vi "get_counter_data.vi"(0 "Counter Settings, Tasks and Data (in)":T1, 5 "error in":errorcluster) -> (14 "Counter Settings, Tasks and Data":T1, 19 "error out":errorcluster)   [LabVIEW 2013]
uses:
  <vilib>/DAQmx/read.llb/DAQmx Read (Counter 1D U32 1Chan NSamp).vi
  <vilib>/DAQmx/miscellaneous.llb/DAQmx Fill In Error Info.vi
panel:
  out "counter data":u32[][](array[numeric])
  out "Last Counters Value":u32[](array[numeric])
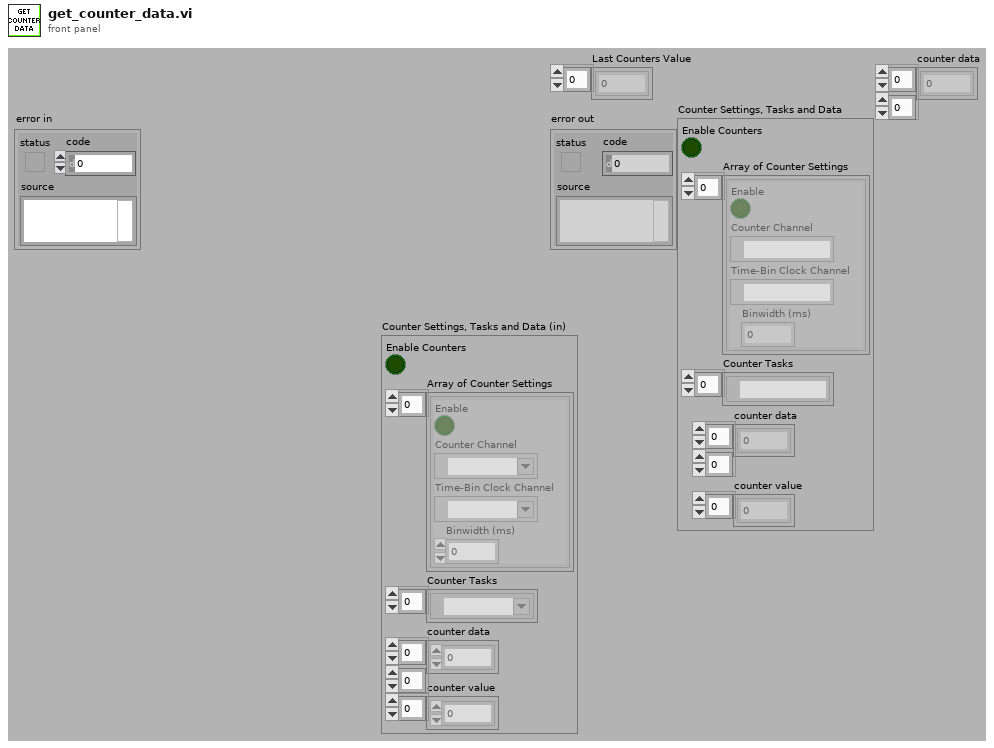
[diagram p1: front panel]
types:
  T1 = cluster{"Enable Counters":bool, "Array of Counter Settings":cluster{"Enable":bool, "Counter Channel":tag, "Time-Bin Clock Channel":tag, "Binwidth (ms)":dbl}[], "Counter Tasks":refnum<k21>[], "counter data":u32[][], "counter value":u32[]}
  T2 = cluster{"Enable":bool, "Counter Channel":tag, "Time-Bin Clock Channel":tag, "Binwidth (ms)":dbl}[]
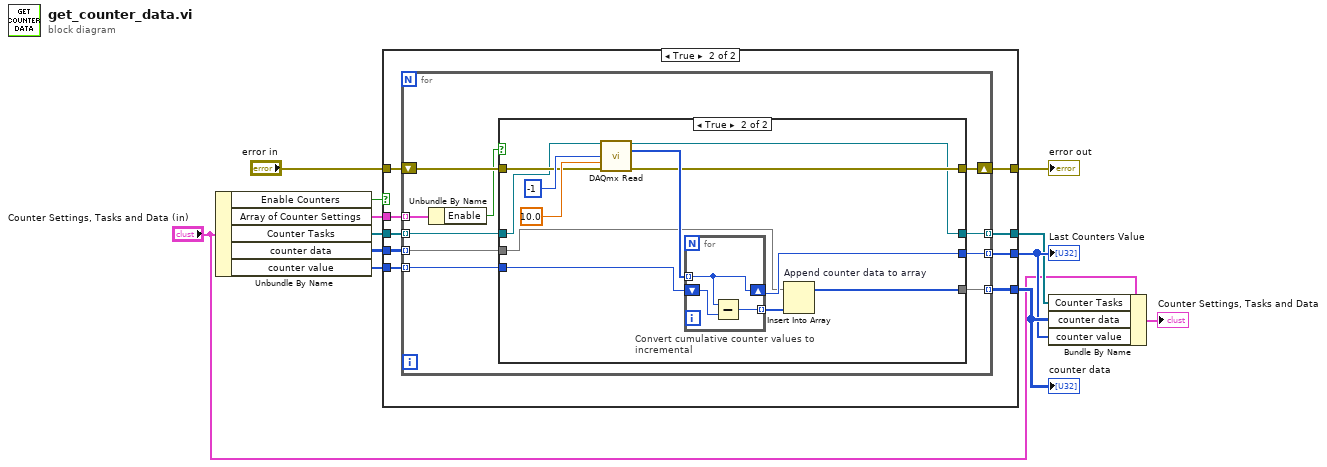
[diagram p0: block diagram]
diagram:
  n1 = Unbundle By Name("Counter Settings, Tasks and Data (in)") -> ("Enable Counters"=w11:bool, "Array of Counter Settings"=w9:T2, "Counter Tasks"=w10:refnum<k21>[], "counter data"=w7:u32[][], "counter value"=w6:u32[])
  n2 = case shown="True" w11 {
    tunnel: w10 -> [w13 w25]
    tunnel: "error in" -> [w16 w24]
    tunnel: w9 -> [_ w23]
    tunnel: [w16 w22] -> w8
    tunnel: [w14 w21] -> w4
    tunnel: w7 -> [w15 w20]
    tunnel: w6 -> [w14 w19]
    tunnel: [w15 w18] -> w5
    tunnel: [w13 w17] -> w2
    frame False {
    }
    frame True {
      n3 = for {
        tunnel: w25 -> [w35] mode=indexing
        tunnel: w23 -> [w33] mode=indexing
        shift-right: [w32] -> w22
        shift-left: w24 -> [w34]
        tunnel: [w30] -> w21 mode=indexing
        tunnel: w20 -> [w29] mode=indexing
        tunnel: w19 -> [w28] mode=indexing
        tunnel: [w27] -> w18 mode=indexing
        tunnel: [w26] -> w17 mode=indexing
        n4 = Unbundle By Name(w33) -> ("Enable"=w31:bool)
        n5 = case shown="True" w31 {
          tunnel: w34 -> [w39 w48]
          tunnel: [w39 w47] -> w32
          tunnel: w35 -> [w36 w45]
          tunnel: [w38 w44] -> w30
          tunnel: w29 -> [w37 w43]
          tunnel: w28 -> [w38 w42]
          tunnel: [w37 w41] -> w27
          tunnel: [w36 w40] -> w26
          frame False {
          }
          frame True {
            n6 = call-poly <vilib>:"DAQmx Read.vi"("task/channels in"=w45, "number of samples per channel"=-1, "timeout"=10.0, "error in"=w48) -> ("task out"=w40:refnum<k21>, "data"=w49:u32[], "error out"=w47:errorcluster)  [unwired: 9 out]
            n7 = for "Convert cumulative counter values to incremental" {
              tunnel: w49 -> [w52] mode=indexing
              shift-right: [w52] -> w44
              shift-left: w42 -> [w54]
              tunnel: [w53] -> w46 mode=indexing
              n8 = Subtract(x=w52, y=w54) -> (x-y=w53:u32)
            }
            n9 = Insert Into Array "Append counter data to array"(array=w43, new element=w46) -> (w41:u32[])  [unwired: 1 in]
          }
        }
      }
    }
  }
  "error out" <- w8
  "Last Counters Value" <- w4
  "counter data" <- w5
  n10 = Bundle By Name(cluster="Counter Settings, Tasks and Data (in)", "Counter Tasks"=w2, "counter data"=w5, "counter value"=w4) -> (→"Counter Settings, Tasks and Data":T1)
